vi "check x and y voltage max.vi"() -> (3 "voltages valid":bool)   [LabVIEW 2017]
doc: "SciScan 1.2 160622"
uses:
  GFG/GFGnumericGet.vi
  GFG/GFGfpRefGet.vi
  GFG/GFG library.lvlib
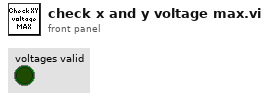
[diagram p1: front panel]
types:
  T1 = enum8{"Enabled", "Disabled", "Disabled and Grayed Out"}
  T2 = cluster{"WaveformChartRef":refnum<vi>, "DigitalRef":refnum<vi>, "ArrayRef":refnum<vi>, "TabControlRef":refnum<vi>, "EnumRef":refnum<vi>, "RingRef":refnum<vi>, "BooleanRef":refnum<vi>, "KnobRef":refnum<vi>, "SlideRef":refnum<vi>, "PathRef":refnum<vi>, "StringRef":refnum<vi>, "ComboBox":refnum<vi>, "WaveformGraphRef":refnum<vi>}
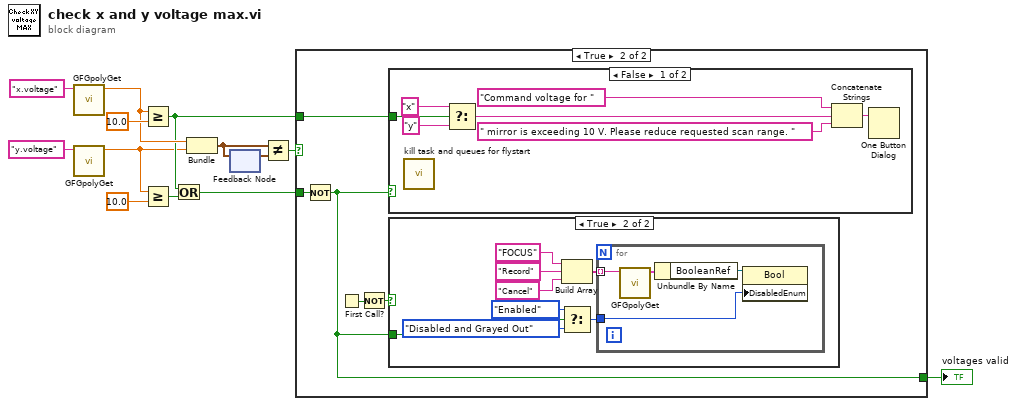
[diagram p0: block diagram]
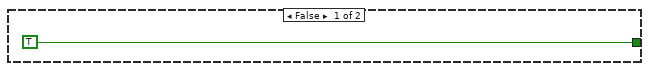
[diagram p2: hidden frame]
diagram:
  n1 = call-poly "GFGpolyGet.vi"("Variable Name in"="x.voltage") -> ("Numeric"=w9:dbl)  [unwired: 8 in, 2 out]
  n2 = call-poly "GFGpolyGet.vi"("Variable Name in"="y.voltage") -> ("Numeric"=w2:dbl)  [unwired: 8 in, 2 out]
  n3 = Greater Or Equal?(x=w9, y=10.0) -> (x >= y?=w4:bool)
  n4 = Greater Or Equal?(x=w2, y=10.0) -> (x >= y?=w1:bool)
  n5 = Or(x=w4, y=w1) -> (x .or. y?=w5:bool)
  n6 = Bundle("Numeric"=w9, "Numeric"=w2) -> (w8:cluster{"Numeric":dbl, "Numeric":dbl})  [unwired: 1 in]
  n7 = feedback-in #1(w8) -> ()
  n8 = feedback #1() -> (w7:cluster{"Numeric":dbl, "Numeric":dbl})  [unwired: 1 in]
  n9 = Not Equal?(x=w8, y=w7) -> (x != y?=w6:bool)
  n10 = case shown="True" w6 {
    tunnel: [TRUE w16] -> w11
    tunnel: w5 -> [_ w17]
    tunnel: w4 -> [_ w15]
    frame False {
    }
    frame True {
      n11 = Not(x=w17) -> (.not. x?=w16:bool)
      n12 = First Call?() -> (First Call?: T/F=w19:bool)
      n13 = Not(x=w19) -> (.not. x?=w18:bool)
      n14 = case shown="False" w16 {
        tunnel: w15 -> [w35 _]
        frame False {
          n15 = call "kill task and queues for flystart.vi"() -> ()  [unwired: 12 in]
          n16 = Select(t="x" ("message"), s=w35, f="y" ("message")) -> (s? t:f=w32:string)
          n17 = Concatenate Strings("Command voltage for " ("message"), w32, " mirror is exceeding 10 V. Please reduce requested scan range. " ("string")) -> (w36:string)
          n18 = One Button Dialog(message=w36) -> ()  [unwired: 1 in, 1 out]
        }
        frame True {
        }
      }
      n19 = case shown="True" w18 {
        tunnel: w16 -> [_ w20]
        frame False {
        }
        frame True {
          n20 = Build Array("FOCUS" ("Variable Name in"), "Record" ("element"), "Cancel" ("element")) -> (w27:string[])
          n21 = Select(t=T1."Enabled" ("Disabled"), s=w20, f=T1."Disabled and Grayed Out" ("Disabled")) -> (s? t:f=w22:T1)
          n22 = for {
            tunnel: w27 -> [w29] mode=indexing
            tunnel: w22 -> [w28]
            n23 = call-poly "GFGpolyGet.vi"("Variable Name in"=w29) -> ("output cluster"=w31:T2)  [unwired: 9 in, 1 out]
            n24 = Unbundle By Name(w31) -> ("BooleanRef"=w30:refnum<vi>)
            n25 = property class="Bool"(reference=w30, "DisabledEnum"=w28) -> ()  [unwired: 1 in, 2 out]
          }
        }
      }
    }
  }
  "voltages valid" <- w11
